vi "Read connected.vi"(8 "error in (no error)":errorcluster, 11 "Socket.Base in":refnum<class "Socket.Base.lvclass">) -> (0 "error out":errorcluster, 2 "connected":bool, 3 "Socket.Base out":refnum<class "Socket.Base.lvclass">)   [LabVIEW 2014, in "Socket.lvlib" / "Socket.Base.lvclass"]
uses:
  Socket.Base.lvclass
  Socket.Base.lvclass/Socket.Base.ctl
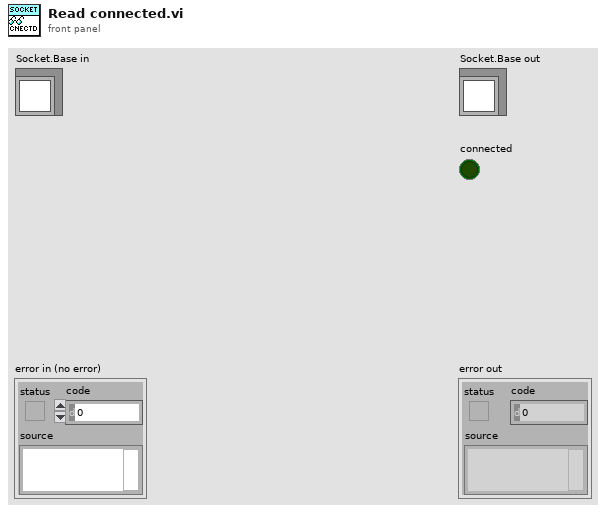
[diagram p1: front panel]
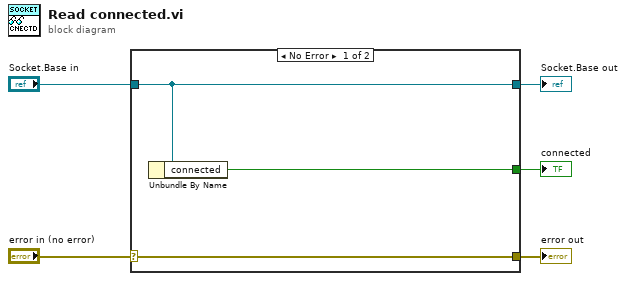
[diagram p0: block diagram]
diagram:
  n1 = case shown="No Error" "error in (no error)" {
    selector: "error in (no error)" -> [w8 w9]
    tunnel: [w8 w9] -> w4
    tunnel: [w7 w10] -> w2
    tunnel: "Socket.Base in" -> [w7 w10]
    tunnel: [w6 _] -> w1
    frame No Error {
      n2 = Unbundle By Name(w7) -> ("connected"=w6:bool)
    }
    frame Error {
    }
  }
  "error out" <- w4
  "Socket.Base out" <- w2
  "connected" <- w1
